vi "motor init connection.vi"(8 "error in (no error)":errorcluster) -> (0 "error out":errorcluster, 3 "Handle Out":i32)   [LabVIEW 2013]
uses:
  private/motor global state actions.ctl
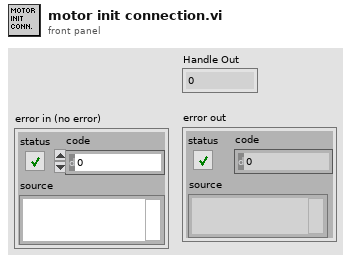
[diagram p1: front panel]
types:
  T1 = typedef "motor global state actions.ctl" = enum16{"set value", "get value", "set angle", "set initialized", "set complete", "set handle", "get handle"}
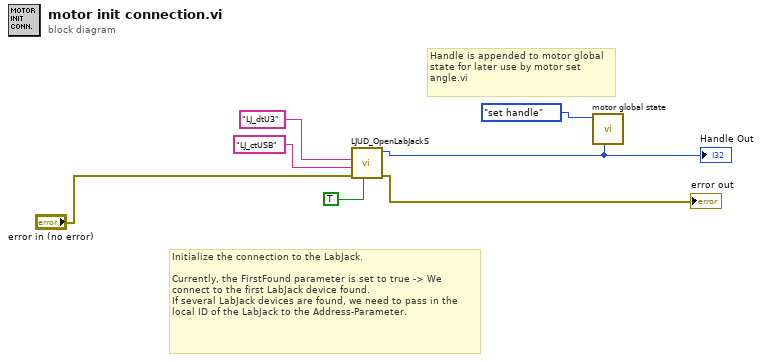
[diagram p0: block diagram]
diagram:
  # "Handle is appended to motor global state for later use by motor set angle.vi"
  # "Initialize the connection to the LabJack.\n\nCurrently, the FirstFound parameter is set to true -> We connect to the first LabJack device found.\nIf several LabJack devices are found, we need to pass in the local ID of the LabJack to the Address-Parameter."
  n1 = call <vilib>:"LJUD_OpenLabJackS.vi"("FirstFound"=TRUE, "error in"="error in (no error)", "ConnectionType"="LJ_ctUSB", "DeviceType"="LJ_dtU3") -> ("error out"=→"error out":errorcluster, "Handle"=w1:i32)  [unwired: 5 in, 1 out]
  "Handle Out" <- w1
  n2 = call "motor global state.vi"("Handle In"=w1, "action"=motor_global_state_actions."set handle" ("Motor FGV actions")) -> ()  [unwired: 8 in, 2 out]
